vi "Teleop.vi"(10 "Match Info":T1={"Autonomous Elapsed Seconds"=0.0, "TeleOp Elapsed Seconds"=0.0, "Disabled Elapsed Seconds"=0.0, "Visited Autonomous"=FALSE, "Visited TeleOp"=FALSE, "Visited Disabled"=FALSE, "Autonomous Settings"={"Autonomous Style"=enum."Independent", "VI Refnum"=refnum}}, 11 "Call Context":T2) -> ()   [LabVIEW 2017]
doc: "This VI is called for each enabled TeleOp packet received from the DS. It is typically used to read from joysticks and other inputs and update I/O or setpoints for timed control loops. It should complete and return within 20 milliseconds or risk missing DS packets."
uses:
  <vilib>/Rock Robotics/WPI/DriverStation/WPI_DriverStationDerivedRobotMode.ctl
  <vilib>/Rock Robotics/WPI/DriverStation/WPI_DriverStationMatch Info.ctl
  <vilib>/Rock Robotics/WPI/Utilities/WPI_GetSetVariantRefNum.vi
  <vilib>/Rock Robotics/Network Tables/NT Write Numeric Array.vi
  <vilib>/Rock Robotics/Network Tables/NT Write Boolean Array.vi
  <vilib>/Rock Robotics/WPI/Joystick/WPI_JoystickArcadeMapping.vi
  Drive/Implementation/gyroNumControl.vi
  <vilib>/FRCT Team# 3937  Breakaway/Memory Library/memLib.lvlib
panel:
  out "Steering Graph":cluster{"X":dbl, "Y":dbl}[](graph)
  out "Throttle Graph":cluster{"X":dbl, "Y":dbl}[](graph)
  out "Drive States":cluster{i16, i16, i16, i16, i16}(graph)
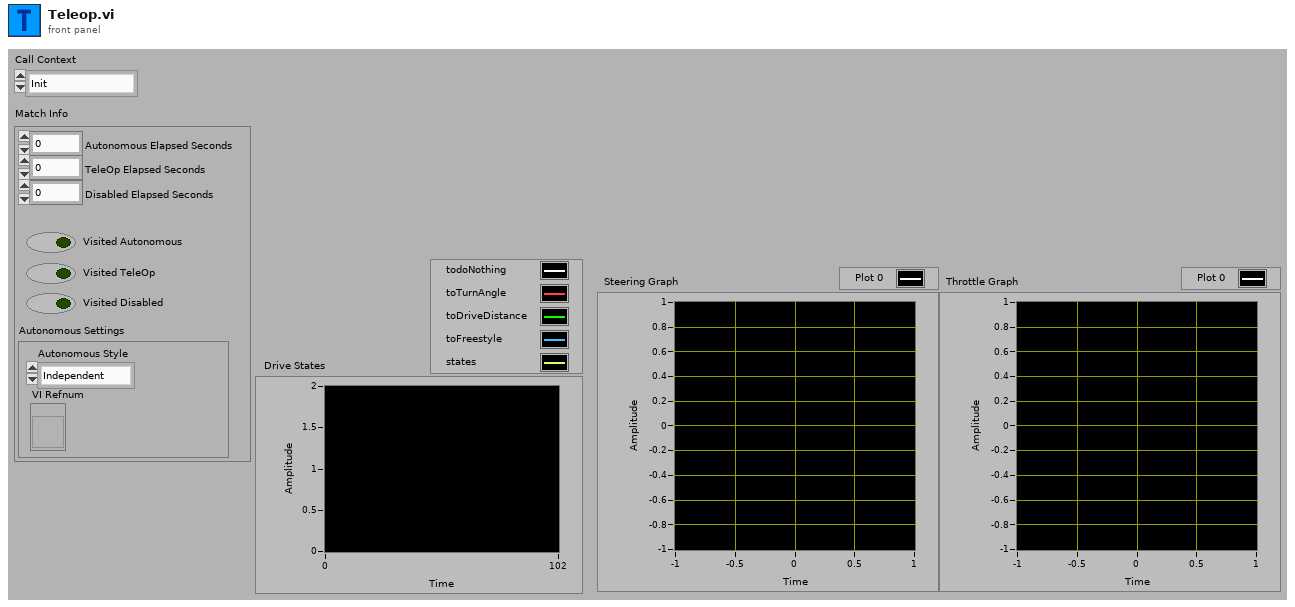
[diagram p1: front panel]
types:
  T1 = typedef "WPI_DriverStationMatch Info.ctl" = cluster{"Autonomous Elapsed Seconds":dbl, "TeleOp Elapsed Seconds":dbl, "Disabled Elapsed Seconds":dbl, "Visited Autonomous":bool, "Visited TeleOp":bool, "Visited Disabled":bool, "Autonomous Settings":cluster{"Autonomous Style":enum16{"Iterative", "Independent"}, "VI Refnum":refnum<vi>}}
  T2 = typedef "WPI_DriverStationDerivedRobotMode.ctl" = enum16{"Init", "Execute", "Stop"}
  T3 = typedef "WPI_JoystickDevRef.ctl" = cluster{"Device":T4}
  T4 = typedef "WPI_JoystickDeviceEnum.ctl" = enum16{"USB 0", "USB 1", "USB 2", "USB 3", "USB 4", "USB 5"}
  T5 = typedef "WPI_SwitchDevRef.ctl" = cluster{"DevStatus":errorcluster, "DIO Channel":T6, "CntIndex":T7, "Normally Closed":bool}
  T6 = typedef "FPGA_DIOChannel.ctl" = enum8{"DIO 0", "DIO 1", "DIO 2", "DIO 3", "DIO 4", "DIO 5", "DIO 6", "DIO 7", "DIO 8", "DIO 9", "DIO MXP 0", "DIO MXP 1", "DIO MXP 2", "DIO MXP 3", "DIO MXP 4", "DIO MXP 5", "DIO MXP 6", "DIO MXP 7", "DIO MXP 8", "DIO MXP 9", "DIO MXP 10", "DIO MXP 11", "DIO MXP 12", "DIO MXP 13", "DIO MXP 14", "DIO MXP 15", "SPI Port CS1", "SPI Port CS2", "SPI Port CS3", "SPI Port MISO", "SPI Port MOSI", "Invalid"}
  T7 = typedef "FPGA_CounterCtrSystemIndex.ctl" = enum8{"Ctr 0", "Ctr 1", "Ctr 2", "Ctr 3", "Ctr 4", "Ctr 5", "Ctr 6", "Ctr 7", "Invalid"}
  T8 = typedef "Drive Operations.ctl" = enum16{"Reserve", "Read Current", "Freestyle", "Drive for Distance", "TurnAngle", "Guided Drive"}
  T9 = typedef "WPI_MotorControlDeviceRef.ctl" = cluster{"DeviceStatus":errorcluster, "Type":T10, "PWM":cluster{"PWM Channel":T11, "DeadBand":T12}, "CAN":cluster{"Device Number":u8, "SetOutput VI Ref":variant, "GetOutput VI Ref":variant, "Enable VI Ref":variant, "Disable VI Ref":variant, "Data":variant}, "Invert":bool, "DIO PWM":cluster{"PWM \"Enable\" Channel":T11, "DIOChannel":T6, "PWM Rate":dbl}}
  T10 = typedef "WPI_MotorControlType.ctl" = enum16{"PWM", "CAN", "DIO PWM"}
  T11 = typedef "FPGA_DIOPWMChannel.ctl" = enum8{"PWM 0", "PWM 1", "PWM 2", "PWM 3", "PWM 4", "PWM 5", "PWM 6", "PWM 7", "PWM 8", "PWM 9", "PWM MXP 0", "PWM MXP 1", "PWM MXP 2", "PWM MXP 3", "PWM MXP 4", "PWM MXP 5", "PWM MXP 6", "PWM MXP 7", "PWM MXP 8", "PWM MXP 9", "Invalid"}
  T12 = typedef "WPI_PWMDeadband.ctl" = cluster{"Name":string, "maxPositivePwm":i32, "minPositivePwm":i32, "centerPwm":i32, "maxNegativePwm":i32, "minNegativePwm":i32, "angularRange":u16}
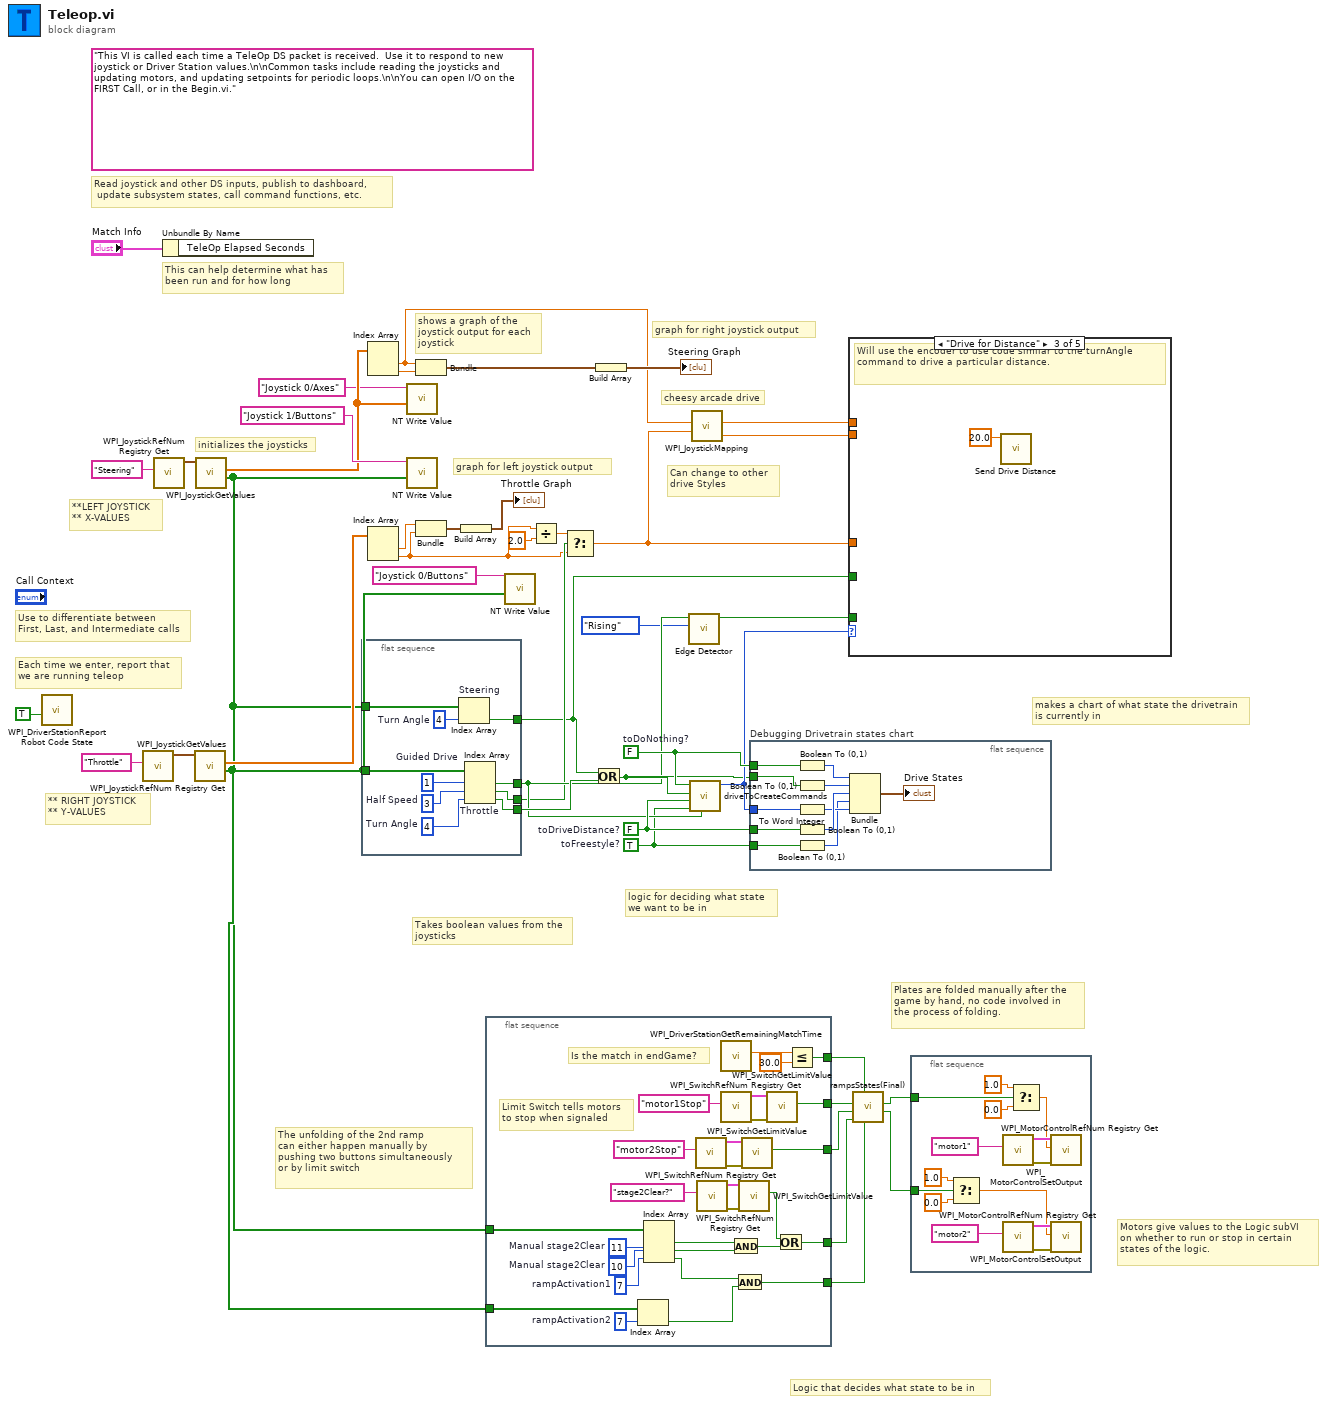
[diagram p0: block diagram]
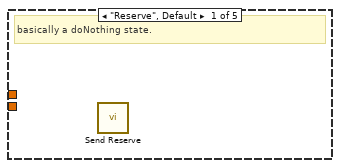
[diagram p2: hidden frame]
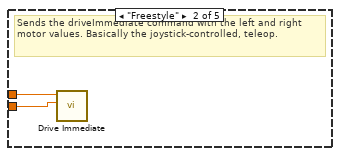
[diagram p3: hidden frame]
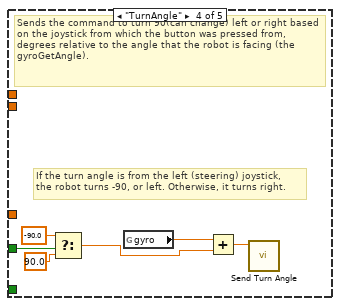
[diagram p4: hidden frame]
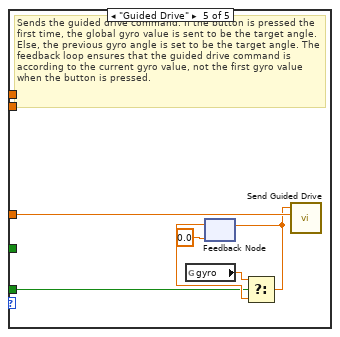
[diagram p5: hidden frame]
diagram:
  w11 = TRUE  # toFreestyle?
  w29 = FALSE  # toDriveDistance?
  w28 = FALSE  # toDoNothing?
  (unwired) "This VI is called each time a TeleOp DS packet is received.  Use it to respond to new joystick or Driver Station values.\n\nCommon tasks include reading the joysticks and updating motors, and updating setpoints for periodic loops.\n\nYou can open I/O on the FIRST Call, or in the Begin.vi."
  # "**LEFT JOYSTICK\n** X-VALUES"
  # "** RIGHT JOYSTICK\n** Y-VALUES"
  # "graph for left joystick output"
  # "graph for right joystick output"
  # "Can change to other\ndrive Styles"
  # "Motors give values to the Logic subVI\non whether to run or stop in certain \nstates of the logic."
  # "The unfolding of the 2nd ramp\ncan either happen manually by \npushing two buttons simultaneously\nor by limit switch"
  # "Logic that decides what state to be in"
  # "Plates are folded manually after the \ngame by hand, no code involved in\nthe process of folding."
  # "logic for deciding what state\nwe want to be in"
  # "cheesy arcade drive"
  # "Takes boolean values from the\njoysticks"
  # "makes a chart of what state the drivetrain\nis currently in"
  # "shows a graph of the\njoystick output for each\njoystick"
  # "initializes the joysticks"
  # "Read joystick and other DS inputs, publish to dashboard,\n update subsystem states, call command functions, etc."
  # "Each time we enter, report that\nwe are running teleop"
  # "Use to differentiate between\nFirst, Last, and Intermediate calls"
  # "This can help determine what has\nbeen run and for how long"
  n1 = call <vilib>:"WPI_DriverStationReport Robot Code State.vi"("TeleOp"=TRUE ("Autonomous")) -> ()  [unwired: 10 in, 1 out]
  n2 = call <vilib>:"WPI_JoystickRefNum Registry Get.vi"("refnum name"="Throttle") -> ("JoystickDevRef"=w22:T3)  [unwired: 1 in, 9 out]
  n3 = call <vilib>:"WPI_JoystickRefNum Registry Get.vi"("refnum name"="Steering") -> ("JoystickDevRef"=w21:T3)  [unwired: 1 in, 9 out]
  n4 = Unbundle By Name("Match Info") -> ()  [unwired: 1 out]
  n5 = call <vilib>:"WPI_JoystickGetValues.vi"("JoystickDevRef"=w22) -> ("Buttons"=w10:bool[], "Axes"=w37:dbl[])  [unwired: 6 in, 3 out]
  n6 = call <vilib>:"WPI_JoystickGetValues.vi"("JoystickDevRef"=w21) -> ("Buttons"=w9:bool[], "Axes"=w40:dbl[])  [unwired: 6 in, 3 out]
  n7 = flat-sequence {
    tunnel: w9 -> [w54]
    tunnel: w10 -> [w48]
    tunnel: [w52] -> w1
    tunnel: [w45] -> w24
    tunnel: [w47] -> w20
    tunnel: [w46] -> w16
    frame #0 {
      w49 = 4  # Turn Angle
      w50 = 3  # Half Speed
      w51 = 1  # Guided Drive
      w53 = 4  # Turn Angle
      n8 = Index Array "Steering"(array=w54, index=w53) -> (element=w52:bool)
      n9 = Index Array "Throttle"(array=w48, index #1=w51, index #2=w50, index #3=w49) -> (element #1=w47:bool, element #2=w46:bool, element #3=w45:bool)
    }
  }
  n10 = Index Array(array=w40) -> (element #1=w17:dbl, element #2=w31:dbl)  [unwired: 2 in]
  n11 = Index Array(array=w37) -> (element #1=w30:dbl, element #2=w14:dbl)  [unwired: 2 in]
  n12 = call-poly <vilib>:"NT Write Value.vi"("Numeric Array"=w40, "Name"="Joystick 0/Axes") -> ()  [unwired: 9 in, 1 out]
  n13 = call-poly <vilib>:"NT Write Value.vi"("Boolean Array"=w9, "Name"="Joystick 1/Buttons") -> ()  [unwired: 9 in, 1 out]
  n14 = Bundle("upper limit"=w17, "upper limit"=w31) -> (w33:cluster{"upper limit":dbl, "upper limit":dbl})  [unwired: 1 in]
  n15 = Bundle("upper limit"=w30, "upper limit"=w14) -> (w35:cluster{"upper limit":dbl, "upper limit":dbl})  [unwired: 1 in]
  n16 = Build Array(w35) -> (→"Throttle Graph":cluster{"upper limit":dbl, "upper limit":dbl}[])
  n17 = flat-sequence {
    tunnel: [w79] -> w7
    tunnel: [w68] -> w4
    tunnel: [w72] -> w8
    tunnel: [w69] -> w5
    tunnel: w10 -> [w65]
    tunnel: w9 -> [w66]
    tunnel: [w58] -> w6
    frame #0 {
      w57 = 11  # Manual stage2Clear
      w67 = 7  # rampActivation1
      w70 = 7  # rampActivation2
      w71 = 10  # Manual stage2Clear
      # "Limit Switch tells motors\nto stop when signaled"
      # "Is the match in endGame?"
      n18 = Index Array(array=w65, index=w70) -> (element=w63:bool)
      n19 = Index Array(array=w66, index #1=w57, index #2=w71, index #3=w67) -> (element #1=w56:bool, element #2=w64:bool, element #3=w62:bool)
      n20 = call <vilib>:"WPI_SwitchRefNum Registry Get.vi"("refnum name"="motor2Stop") -> ("error out"=w60:errorcluster, "SwitchDevRef"=w61:T5)  [unwired: 9 in]
      n21 = call <vilib>:"WPI_SwitchRefNum Registry Get.vi"("refnum name"="stage2Clear?") -> ("error out"=w77:errorcluster, "SwitchDevRef"=w78:T5)  [unwired: 9 in]
      n22 = call <vilib>:"WPI_DriverStationGetRemainingMatchTime.vi"() -> ("Match Time(s)"=w74:sgl)  [unwired: 10 in, 1 out]
      n23 = call <vilib>:"WPI_SwitchRefNum Registry Get.vi"("refnum name"="motor1Stop") -> ("error out"=w80:errorcluster, "SwitchDevRef"=w81:T5)  [unwired: 9 in]
      n24 = And(x=w56, y=w64) -> (x .and. y?=w55:bool)
      n25 = And(x=w62, y=w63) -> (x .and. y?=w69:bool)
      n26 = call <vilib>:"WPI_SwitchGetLimitValue.vi"("error in (no error)"=w77, "SwitchDevRef"=w78) -> ("Switch Pressed"=w75:bool)  [unwired: 7 in, 2 out]
      n27 = call <vilib>:"WPI_SwitchGetLimitValue.vi"("error in (no error)"=w60, "SwitchDevRef"=w61) -> ("Switch Pressed"=w58:bool)  [unwired: 7 in, 2 out]
      n28 = call <vilib>:"WPI_SwitchGetLimitValue.vi"("error in (no error)"=w80, "SwitchDevRef"=w81) -> ("Switch Pressed"=w79:bool)  [unwired: 7 in, 2 out]
      n29 = Or(x=w75, y=w55) -> (x .or. y?=w68:bool)
      n30 = Less Or Equal?(x=w74, y=sgl 30.0 ("Match Time(s)")) -> (x <= y?=w72:bool)
    }
  }
  n31 = call-poly <vilib>:"NT Write Value.vi"("Boolean Array"=w10, "Name"="Joystick 0/Buttons") -> ()  [unwired: 9 in, 1 out]
  n32 = Divide(x=w14, y=2.0) -> (x/y=w13:dbl)
  n33 = Select(t=w13, s=w16, f=w14) -> (s? t:f=w12:dbl)
  n34 = Or(x=w1, y=w24) -> (x .or. y?=w23:bool)
  n35 = Build Array(w33) -> (→"Steering Graph":cluster{"upper limit":dbl, "upper limit":dbl}[])
  n36 = call <vilib>:"Edge Detector.vi"("Mode"=enum16{"Rising", "Falling", "Any"}."Rising", "Input"=w20) -> ("Output"=w18:bool)  [unwired: 9 in]
  n37 = call "driveToCreateCommands.vi"("toGuidedDrive"=w20, "toFreestyle"=w11, "toDriveDistance"=w29, "toTurnAngle"=w23, "toReserve"=w28) -> ("Current State"=w27:T8)  [unwired: 6 in]
  n38 = call-poly <vilib>:"WPI_JoystickMapping.vi"("Y axis value"=w12, "X axis value"=w17) -> ("Right Motor Value"=w25:dbl, "Left Motor Value"=w26:dbl)  [unwired: 8 in]
  n39 = flat-sequence "Debugging Drivetrain states chart" {
    tunnel: w29 -> [w93]
    tunnel: w23 -> [w92]
    tunnel: w28 -> [w91]
    tunnel: w27 -> [w85]
    tunnel: w11 -> [w84]
    frame #0 {
      n40 = Boolean To (0,1)(Boolean=w91) -> (0, 1=w88:i16)
      n41 = Boolean To (0,1)(Boolean=w92) -> (0, 1=w89:i16)
      n42 = To Word Integer(number=w85) -> (16bit integer=w86:i16)
      n43 = Boolean To (0,1)(Boolean=w93) -> (0, 1=w90:i16)
      n44 = Boolean To (0,1)(Boolean=w84) -> (0, 1=w83:i16)
      n45 = Bundle(w88, w89, w90, w83, w86) -> (→"Drive States":cluster{i16, i16, i16, i16, i16})  [unwired: 1 in]
    }
  }
  n46 = case shown="\"Drive for Distance\"" w27 {
    tunnel: w26 -> [_ w95 _ _ _]
    tunnel: w25 -> [_ w94 _ _ _]
    tunnel: w12 -> [_ _ _ _ w108]
    tunnel: w18 -> [_ _ _ _ w103]
    tunnel: w1 -> [_ _ _ w100 _]
    frame "Reserve", Default {
      # "basically a doNothing state."
      n47 = call "Send Reserve.vi"() -> ()  [unwired: 10 in, 2 out]
    }
    frame "Freestyle" {
      # "Sends the driveImmediate command with the left and right motor values. Basically the joystick-controlled, teleop."
      n48 = call "Drive Immediate.vi"("Right Setpoint"=w94, "Left Setpoint"=w95) -> ()  [unwired: 9 in, 1 out]
    }
    frame "Drive for Distance" {
      # "Will use the encoder to use code similar to the turnAngle command to drive a particular distance."
      n49 = call "Send Drive Distance.vi"("Target Distance"=20.0) -> ()  [unwired: 9 in, 2 out]
    }
    frame "TurnAngle" {
      # "If the turn angle is from the left (steering) joystick, \nthe robot turns -90, or left. Otherwise, it turns right."
      # "Sends the command to turn 90(can change) left or right based on the joystick from which the button was pressed from, degrees relative to the angle that the robot is facing (the gyroGetAngle)."
      n50 = Select(t=-90.0, s=w100, f=90.0) -> (s? t:f=w97:dbl)
      n51 = global read "gyroNumControl.vi" "gyro"() -> (w102:dbl)
      n52 = Add(x=w102, y=w97) -> (x+y=w101:dbl)
      n53 = call "Send Turn Angle.vi"("Target Angle"=w101) -> ()  [unwired: 9 in, 2 out]
    }
    frame "Guided Drive" {
      # "Sends the guided drive command. If the button is pressed the first time, the global gyro value is sent to be the target angle. Else, the previous gyro angle is set to be the target angle. The feedback loop ensures that the guided drive command is according to the current gyro value, not the first gyro value when the button is pressed."
      n54 = global read "gyroNumControl.vi" "gyro"() -> (w104:dbl)
      n55 = feedback #1(0.0 ("Angle")) -> (w105:dbl)
      n56 = Select(t=w104, s=w103, f=w105) -> (s? t:f=w107:dbl)
      n57 = feedback-in #1(w107) -> ()
      n58 = call "Send Guided Drive.vi"("Y-value"=w108, "Target Angle"=w107) -> ()  [unwired: 8 in, 2 out]
    }
  }
  n59 = call "rampsStates(Final).vi"("buttonsPushed?"=w5, "endGame?"=w8, "stage2Clear?"=w4, "motor2Stop"=w6, "motor1Stop"=w7) -> ("motor2"=w2:bool, "motor1"=w3:bool)  [unwired: 5 in]
  n60 = flat-sequence {
    tunnel: w3 -> [w110]
    tunnel: w2 -> [w109]
    frame #0 {
      n61 = Select(t=1.0, s=w109, f=0.0) -> (s? t:f=w113:dbl)
      n62 = call <vilib>:"WPI_MotorControlRefNum Registry Get.vi"("refnum name"="motor1") -> ("error out"=w120:errorcluster, "MotorControlDevRef"=w121:T9)  [unwired: 9 in]
      n63 = call <vilib>:"WPI_MotorControlRefNum Registry Get.vi"("refnum name"="motor2") -> ("error out"=w114:errorcluster, "MotorControlDevRef"=w115:T9)  [unwired: 9 in]
      n64 = Select(t=1.0, s=w110, f=0.0) -> (s? t:f=w119:dbl)
      n65 = call <vilib>:"WPI_MotorControlSetOutput.vi"("error in (no error)"=w120, "Output"=w119, "MotorControlDevRef"=w121) -> ()  [unwired: 6 in, 3 out]
      n66 = call <vilib>:"WPI_MotorControlSetOutput.vi"("error in (no error)"=w114, "Output"=w113, "MotorControlDevRef"=w115) -> ()  [unwired: 6 in, 3 out]
    }
  }
